vi "generate floor and ceiling point.vi"(10 "Game Parameters":T3={"Upper Limit (m)"=100.0, "Lower Limit (m)"=0.0, "Obstacle time"=20.0, "Obstacle length"=10.0, "fuel decrement"=0.5, "Fuel time"=100.0, "fuel amount"=50.0, "Fuel range"=10, "Death range"=5, "Terrain slope"=35.0, "Speed (km/hr)"=150.0, "Time step (ms)"=30, "Gravity"=-9.81, "Date"="11/03/2016", "High scores path"=path "C:/Users/lz2/Code/LabVIEW/Helicopter/hi scores.txt", "Difficulty"=enum."Normal", "Headstart"=30}, 11 "Arrays and Heights":T1={"Score Array"=[], "Lowest high score"=0.0, "Score"=0.0, "Ceiling"=0.0, "Floor"=0.0, "Ceiling Array"=[], "Floor array"=[], "Helicopter height"=0.0, "Helicopter array"=[], "Fuel"=300.0, "Fuel array"=[], "fuel counter"=0, "obstacle counter"=0, "Obstacle array"=[], "helicopter v_0"=0.0, "helicopter a_0"=0.0, "Obstacle height"=300.0}) -> (3 "Arrays and values":T1={"Score Array"=[], "Lowest high score"=0.0, "Score"=0.0, "Ceiling"=0.0, "Floor"=0.0, "Ceiling Array"=[], "Floor array"=[], "Helicopter height"=0.0, "Helicopter array"=[], "Fuel"=300.0, "Fuel array"=[], "fuel counter"=0, "obstacle counter"=0, "Obstacle array"=[], "helicopter v_0"=0.0, "helicopter a_0"=0.0, "Obstacle height"=300.0})   [LabVIEW 2017]
uses:
  controls/arrays and heights.ctl
  controls/scores.ctl
  controls/game parameters.ctl
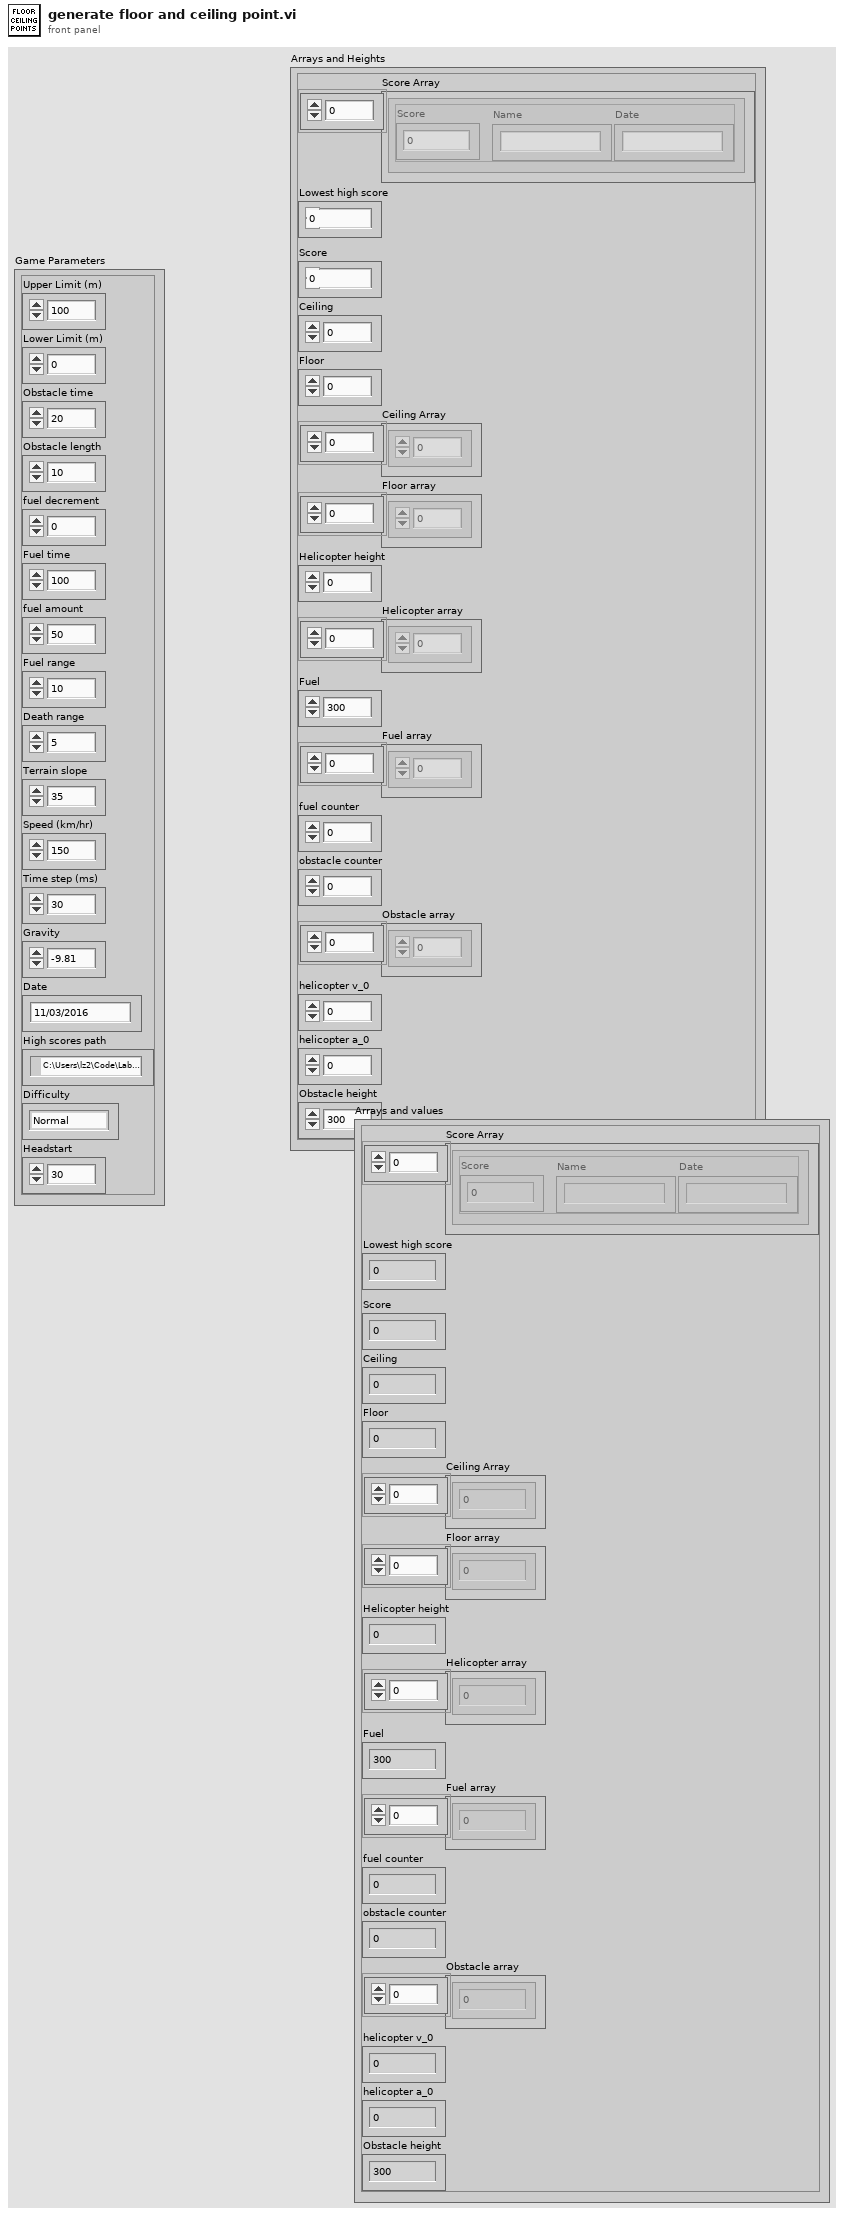
[diagram p1: front panel]
types:
  T1 = typedef "arrays and heights.ctl" = cluster{"Score Array":T2[], "Lowest high score":dbl, "Score":dbl, "Ceiling":dbl, "Floor":dbl, "Ceiling Array":dbl[], "Floor array":dbl[], "Helicopter height":dbl, "Helicopter array":dbl[], "Fuel":dbl, "Fuel array":dbl[], "fuel counter":i32, "obstacle counter":i32, "Obstacle array":dbl[], "helicopter v_0":dbl, "helicopter a_0":dbl, "Obstacle height":dbl}
  T2 = typedef "scores.ctl" = cluster{"Score":dbl, "Name":string, "Date":string}
  T3 = typedef "game parameters.ctl" = cluster{"Upper Limit (m)":dbl, "Lower Limit (m)":dbl, "Obstacle time":dbl, "Obstacle length":dbl, "fuel decrement":dbl, "Fuel time":dbl, "fuel amount":dbl, "Fuel range":i32, "Death range":i32, "Terrain slope":dbl, "Speed (km/hr)":dbl, "Time step (ms)":u32, "Gravity":dbl, "Date":string, "High scores path":path, "Difficulty":enum16{"Easy", "Normal", "Hard"}, "Headstart":u32}
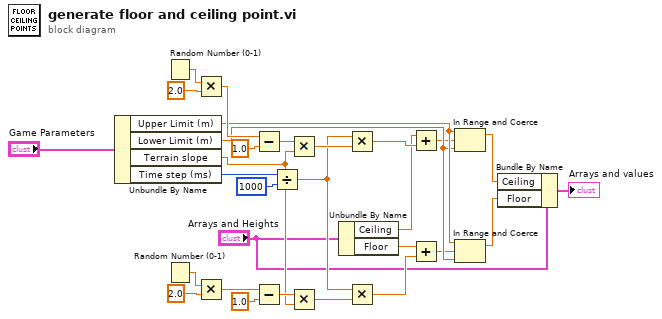
[diagram p0: block diagram]
diagram:
  n1 = Unbundle By Name("Game Parameters") -> ("Upper Limit (m)"=w6:dbl, "Lower Limit (m)"=w5:dbl, "Terrain slope"=w12:dbl, "Time step (ms)"=w10:u32)
  n2 = Random Number (0-1)() -> (number: 0 to 1=w25:dbl)
  n3 = Random Number (0-1)() -> (number: 0 to 1=w19:dbl)
  n4 = Multiply(x=w25, y=2.0) -> (x*y=w27:dbl)
  n5 = Multiply(x=w19, y=2.0) -> (x*y=w17:dbl)
  n6 = Subtract(x=w27, y=1.0) -> (x-y=w24:dbl)
  n7 = Subtract(x=w17, y=1.0) -> (x-y=w20:dbl)
  n8 = Divide(x=w10, y=u32 1000) -> (x/y=w9:dbl)
  n9 = Multiply(x=w24, y=w12) -> (x*y=w23:dbl)
  n10 = Multiply(x=w20, y=w12) -> (x*y=w21:dbl)
  n11 = Unbundle By Name("Arrays and Heights") -> ("Ceiling"=w15:dbl, "Floor"=w14:dbl)
  n12 = Multiply(x=w9, y=w23) -> (x*y=w29:dbl)
  n13 = Multiply(x=w9, y=w21) -> (x*y=w22:dbl)
  n14 = Add(x=w15, y=w29) -> (x+y=w3:dbl)
  n15 = Add(x=w14, y=w22) -> (x+y=w4:dbl)
  n16 = In Range and Coerce(upper limit=w6, x=w3, lower limit=w5) -> (coerced(x)=w2:dbl)  [unwired: 1 out]
  n17 = In Range and Coerce(upper limit=w6, x=w4, lower limit=w5) -> (coerced(x)=w1:dbl)  [unwired: 1 out]
  n18 = Bundle By Name(cluster="Arrays and Heights", "Ceiling"=w2, "Floor"=w1) -> (→"Arrays and values":T1)
